vi "Create Failure Response.vi"() -> (2 "output cluster":T1)   [LabVIEW 2024]
uses:
  Private/Typedefs/Messages/JSON Response.ctl
  Sift Client.lvlib
  Private/Typedefs/Messages/Reason.ctl
panel:
  in  "Reason":T2
  in  "JSON Response":T1
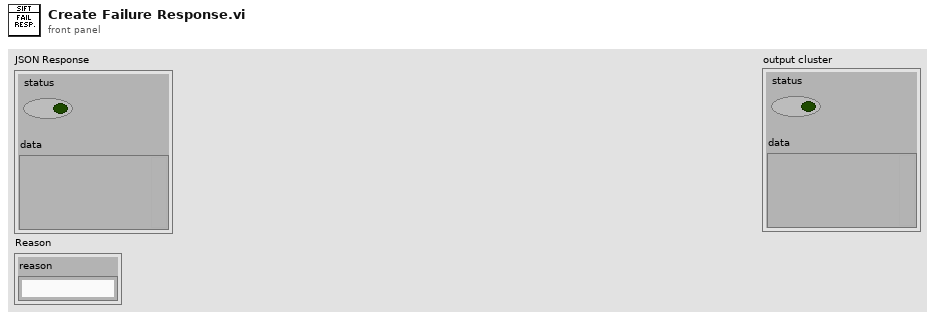
[diagram p1: front panel]
types:
  T1 = typedef "Sift Client.lvlib/JSON Response.ctl" = cluster{"status":bool, "data":variant}
  T2 = typedef "Sift Client.lvlib/Reason.ctl" = cluster{"reason":string}
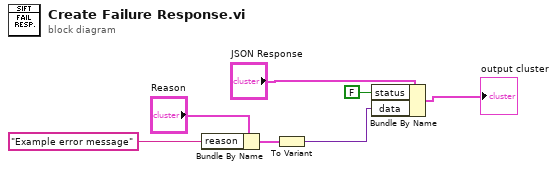
[diagram p0: block diagram]
diagram:
  n1 = Bundle By Name(cluster="Reason", "reason"="Example error message" ("ingestion_config_id")) -> (w4:T2)
  n2 = To Variant(anything=w4) -> (Variant=w3:variant)
  n3 = Bundle By Name(cluster="JSON Response", "status"=FALSE, "data"=w3) -> (→"output cluster":T1)
